vi "generatore_stringa_casuale.vi"() -> (2 "stringa":string)   [LabVIEW 2013]
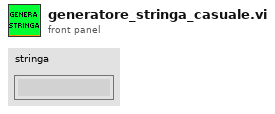
[diagram p1: front panel]
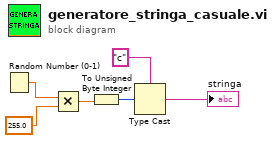
[diagram p0: block diagram]
diagram:
  n1 = Random Number (0-1)() -> (number: 0 to 1=w6:dbl)
  n2 = Multiply(x=w6, y=255.0) -> (x*y=w4:dbl)
  n3 = To Unsigned Byte Integer(number=w4) -> (unsigned 8bit integer=w3:u8)
  n4 = Type Cast(type="c", x=w3) -> (*(type *) &x=→"stringa":string)
